vi "test_Add Command_Invalid Command or Response Ref Error.vi"(8 "error in (no error)":errorcluster, 11 "TestCase in":refnum<class "Instrument Addon Scripting API Messages Unit Tests.lvclass">) -> (0 "error out":errorcluster, 3 "TestCase out":refnum<class "Instrument Addon Scripting API Messages Unit Tests.lvclass">)   [LabVIEW 2020, in "Instrument Addon Scripting API Messages Unit Tests.lvclass"]
uses:
  Instrument Addon Scripting API Messages Unit Tests.lvclass
  APIs/Scripting API/TypeDefs/Command Settings.ctl
  <vilib>/NI VeriStand/Custom Device API/Custom Device Item Ref.ctl
  APIs/Scripting API/TypeDefs/Padding.ctl
  Instrument Addon Scripting API Messages Unit Tests.lvclass/Instrument Addon Scripting API Messages Unit Tests.ctl
  Addon/Addon Shared/SubVIs/Constants.vi
  <vilib>/NI/NI VeriStand Advanced SysDef API/_SubVIs/SysDef.Search.GUID.vi
  <vilib>/addons/_JKI Toolkits/VI Tester/TestCase.llb/TestCase.lvclass
  <vilib>/NI VeriStand/Custom Device API/Custom Device API.lvlib
  APIs/Scripting API/Instrument Addon Scripting API.lvlib
  Addon/Addon Shared/Instrument Addon Shared.lvlib
  <vilib>/NI/NI VeriStand Advanced SysDef API/SysDef API/Advanced System Definition.lvlib
  C:/Program Files (x86)/National Instruments/LabVIEW 2020/vi.lib/addons/_JKI Toolkits/VI Tester/TestCase.llb/TestCase.lvclass
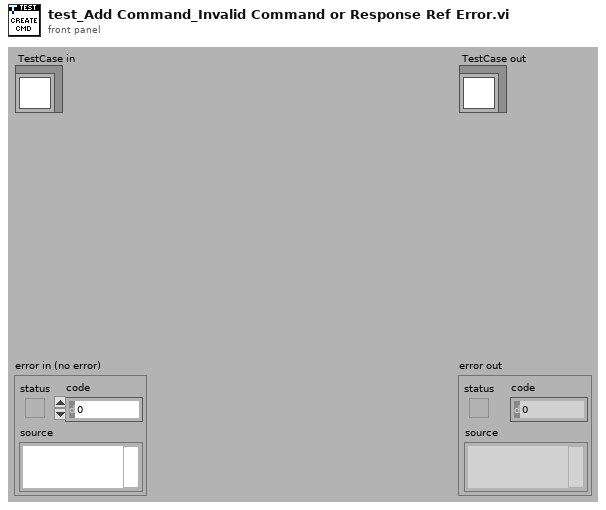
[diagram p1: front panel]
types:
  T1 = typedef "Instrument Addon Scripting API.lvlib/Command Settings.ctl" = cluster{"Command Format":string, "Linked Channels":cluster{"Variable Name":string, "Channel Ref in":T2}[], "Use Padding?":bool, "Padding":T3}
  T2 = typedef "Custom Device API.lvlib/Custom Device Item Ref.ctl" = u64
  T3 = typedef "Instrument Addon Scripting API.lvlib/Padding.ctl" = cluster{"Pad Value":u8, "Length":u32}
  T4 = typedef "Instrument Addon Scripting API.lvlib/Linked Channel.ctl" = cluster{"Variable Name":string, "Channel Refnum":T2}
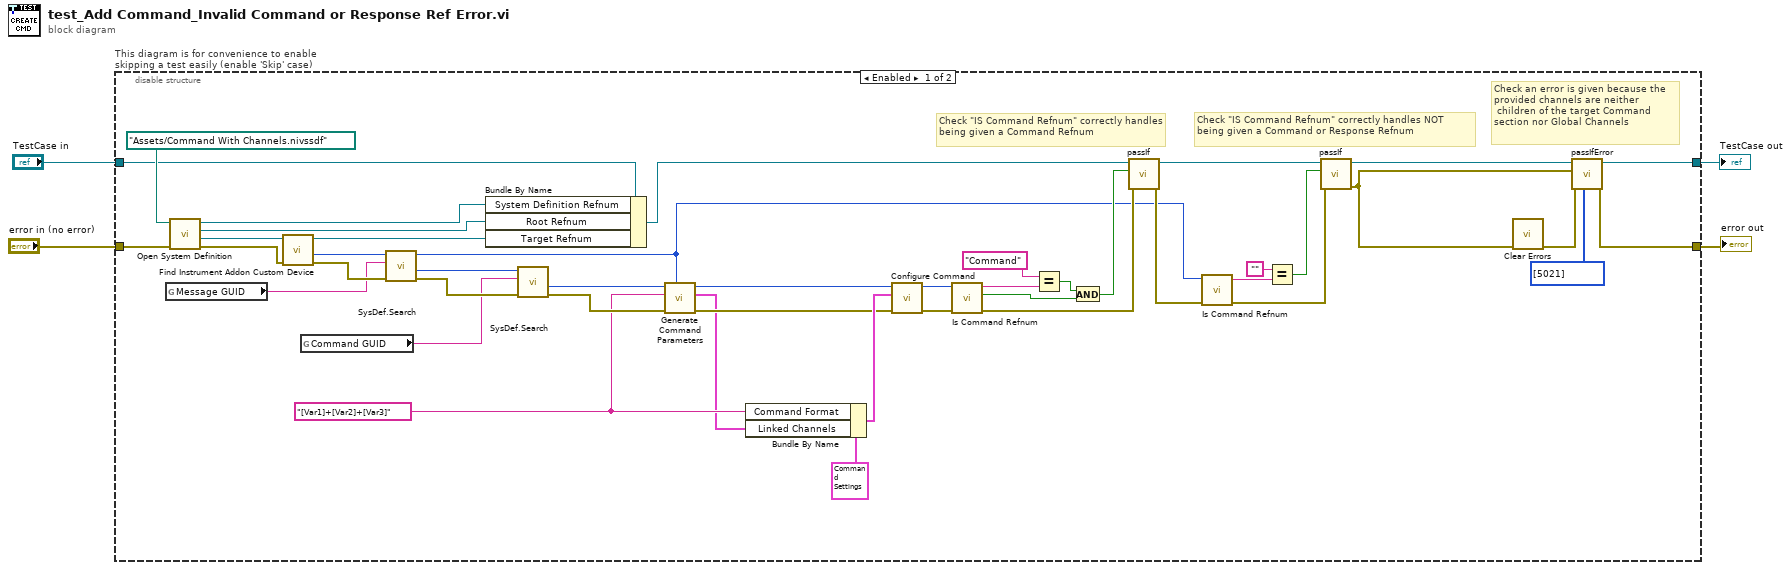
[diagram p0: block diagram]
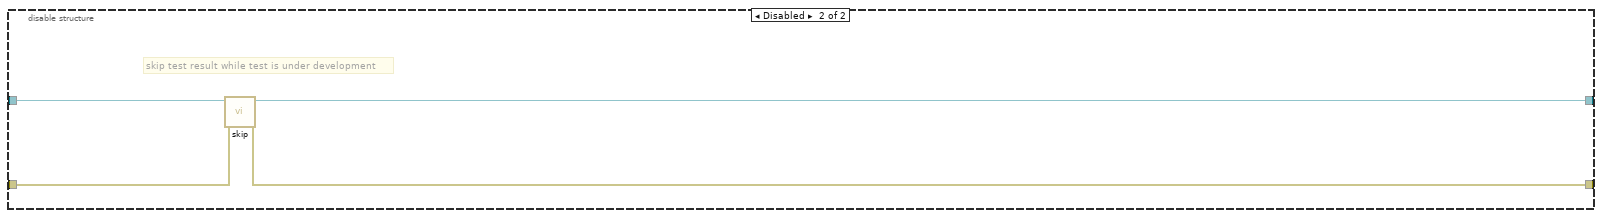
[diagram p2: hidden frame]
diagram:
  n1 = disable-structure "This diagram is for convenience to enable skipping a test easily (enable 'Skip' case)" shown="Enabled" {
    disable-tunnel: "TestCase in" -> [w22 w52]
    disable-tunnel: [w45 w50] -> w1
    disable-tunnel: [w46 w51] -> w3
    disable-tunnel: "error in (no error)" -> [w47 w49]
    frame Enabled {
      w7 = "[Var1]+[Var2]+[Var3]" ("Command Format")
      # "Check \"IS Command Refnum\" correctly handles NOT being given a Command or Response Refnum"
      # "Check \"IS Command Refnum\" correctly handles being given a Command Refnum"
      # "Check an error is given because the provided channels are neither\n children of the target Command section nor Global Channels"
      n2 = global read "Constants.vi" "Message GUID"() -> (w41:string)
      n3 = call "Open System Definition.vi"("error in (no error)"=w47, "System Definition File"=path "Assets/Command With Channels.nivssdf" ("SDF file")) -> ("error out"=w43:errorcluster, "Target Refnum"=w44:refnum<k24>, "Root Refnum"=w19:refnum<k24>, "System Definition Refnum"=w20:refnum<k24>)  [unwired: 6 in]
      n4 = call "Find Instrument Addon Custom Device.vi"("error in"=w43, "target in"=w44) -> ("error out"=w42:errorcluster, "NodeID"=w39:u64, "target out"=w18:refnum<k24>)  [unwired: 7 in]
      n5 = global read "Constants.vi" "Command GUID"() -> (w12:string)
      n6 = call-poly <vilib>:"SysDef.Search.vi"("error in (no error)"=w42, "GUID"=w41, "nodeID"=w39) -> ("error out"=w13:errorcluster, "Value out"=w14:u64, "nodeID out"=w6:u64)  [unwired: 5 in, 1 out]
      n7 = Bundle By Name(cluster=w22, "System Definition Refnum"=w20, "Root Refnum"=w19, "Target Refnum"=w18) -> (w21:refnum<class "Instrument Addon Scripting API Messages Unit Tests.lvclass">)
      n8 = call-poly <vilib>:"SysDef.Search.vi"("error in (no error)"=w13, "GUID"=w12, "nodeID"=w14) -> ("error out"=w9:errorcluster, "Value out"=w11:u64)  [unwired: 5 in, 2 out]
      n9 = call "Generate Command Parameters.vi"("Instrument Addon Refnum in"=w6, "Error In"=w9, "Command String"=w7, "Command Channel in"=w11) -> ("Error Out"=w8:errorcluster, "Linked Channels"=w5:T4[], "Command Channel out"=w10:T2)  [unwired: 4 in, 1 out]
      n10 = Bundle By Name(cluster=T1 {"Command Format"="[Var1]+[Var2]", "Linked Channels"=[{"Variable Name"="Var1", "Channel Ref in"=32}, {"Variable Name"="Var2", "Channel Ref in"=33}], "Use Padding?"=FALSE, "Padding"={"Pad Value"=0, "Length"=0}} ("Settings"), "Command Format"=w7, "Linked Channels"=w5) -> (w15:T1)
      n11 = call "Configure Command.vi"("error in (no error)"=w8, "settings"=w15, "command refnum in"=w10) -> ("error out"=w17:errorcluster, "command refnum out"=w16:T2)  [unwired: 7 in]
      n12 = call "Is Command Refnum.vi"("error in (no error)"=w17, "Command/Response Refnum in"=w16) -> ("error out"=w36:errorcluster, "Is Command?"=w32:bool, "Command/Response out"=w35:string)  [unwired: 7 in]
      n13 = Equal?(x="Command", y=w35) -> (x = y?=w33:bool)
      n14 = And(x=w33, y=w32) -> (x .and. y?=w31:bool)
      n15 = call-dynamic "passIf.vi"("error in (no error)"=w36, "pass"=w31, "TestCase in"=w21) -> ("error out"=w30:errorcluster, "TestCase out"=w24:refnum<class "Instrument Addon Scripting API Messages Unit Tests.lvclass">)  [unwired: 7 in]
      n16 = call "Is Command Refnum.vi"("error in (no error)"=w30, "Command/Response Refnum in"=w6) -> ("error out"=w26:errorcluster, "Command/Response out"=w28:string)  [unwired: 7 in, 1 out]
      n17 = Equal?(x="", y=w28) -> (x = y?=w27:bool)
      n18 = call-dynamic "passIf.vi"("error in (no error)"=w26, "pass"=w27, "TestCase in"=w24) -> ("error out"=w25:errorcluster, "TestCase out"=w23:refnum<class "Instrument Addon Scripting API Messages Unit Tests.lvclass">)  [unwired: 7 in]
      n19 = call <vilib>:"Clear Errors.vi"("error in (no error)"=w25) -> ("error out"=w37:errorcluster)  [unwired: 5 in, 1 out]
      n20 = call-dynamic "passIfError.vi"("passing error codes (default = any error code)"=i32[] [5021], "error in (no error)"=w37, "error"=w25, "TestCase in"=w23) -> ("error out"=w46:errorcluster, "TestCase out"=w45:refnum<class "Instrument Addon Scripting API Messages Unit Tests.lvclass">)  [unwired: 6 in]
    }
    frame Disabled {
      # "skip test result while test is under development"
      n21 = call <vilib>:"skip.vi"("error in (no error)"=w49, "TestCase in"=w52) -> ("error out"=w51:errorcluster, "TestCase out"=w50:refnum<class "Instrument Addon Scripting API Messages Unit Tests.lvclass">)  [unwired: 8 in]
    }
  }
  "error out" <- w3
  "TestCase out" <- w1
